vi "network-adapter_verify.vi"(8 "error in (no error)":errorcluster, 11 "adapter_name":string) -> (0 "error out":errorcluster, 2 "found?":bool, 3 "connected?":bool)   [LabVIEW 2015, in "lv-bin-windows.lvlib" / "v1.lvlib"]
uses:
  v1.lvlib
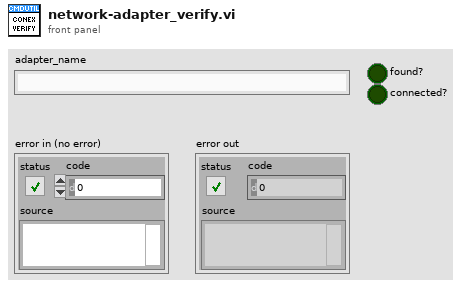
[diagram p1: front panel]
types:
  T1 = typedef "lv-bin-windows.lvlib/v1.lvlib/adapter.ctl" = cluster{"adapter_name":string, "physical_address":string, "ipv4_address":string, "subnet_mask":string, "default_gateway":string, "description":string, "media_state":string}
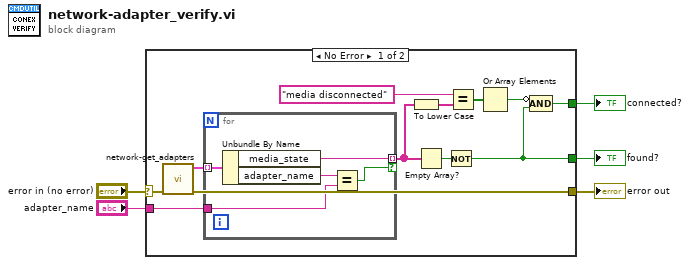
[diagram p0: block diagram]
diagram:
  n1 = case shown="No Error" "error in (no error)" {
    selector: "error in (no error)" -> [w16 w23]
    tunnel: "adapter_name" -> [w14 _]
    tunnel: [w11 _] -> w3
    tunnel: [w6 w23] -> w2
    tunnel: [w17 _] -> w1
    frame No Error {
      n2 = call "network-get_adapters.vi"("error in (no error)"=w16) -> ("error out"=w6:errorcluster, "adapter []"=w15:T1[])  [unwired: 9 in]
      n3 = for {
        tunnel: w15 -> [w22] mode=indexing
        tunnel: w14 -> [w21]
        tunnel: [w19] -> w13 mode=indexing if=w18
        n4 = Unbundle By Name(w22) -> ("media_state"=w19:string, "adapter_name"=w20:string)
        n5 = Equal?(x=w20, y=w21) -> (x = y?=w18:bool)
      }
      n6 = To Lower Case(string=w13) -> (all lower case string=w10:string[])
      n7 = Empty Array?(array=w13) -> (empty?=w12:bool)
      n8 = Not(x=w12) -> (.not. x?=w11:bool)
      n9 = Equal?(x="media disconnected", y=w10) -> (x = y?=w8:bool[])
      n10 = Or Array Elements(Boolean array=w8) -> (logical OR=w7:bool)
      n11 = Compound Arithmetic op=AND(invert w7, w11) -> (w17:bool)
    }
    frame Error {
    }
  }
  "error out" <- w2
  "found?" <- w3
  "connected?" <- w1
